vi "prueba_bloques.vi"() -> ()   [LabVIEW 2019]
uses:
  <vilib>/imath/engines/lvmath2/RunTimeEngine/Managers/WorkSpace/UID Generator.vi
  <vilib>/imath/engines/lvmath2/RunTimeEngine/IndexRead/NIMS V(S).vi
  <instcachedir>/0/NIMS V(S)_0488751826AF41519A22953C041130DC.lvgen/NIMS V(S)_0488751826AF41519A22953C041130DC_000.vi
  <vilib>/imath/engines/lvmath2/RunTimeEngine/BuiltInFunctions/atan2/NIMS_atan2.vi
  <instcachedir>/0/NIMS_atan2_A91AA4A7D42247EDBE8F76DB99AF04A4.lvgen/NIMS_atan2_A91AA4A7D42247EDBE8F76DB99AF04A4_000.vi
  <vilib>/imath/engines/lvmath2/RunTimeEngine/ErrorHandling/NIMS_Create Error From Enums.vi
  <vilib>/imath/engines/lvmath2/RunTimeEngine/ArithmeticOperatorToken/NIMS_ArithmeticOperator_power(S).vi
  <instcachedir>/0/NIMS_ArithmeticOperator_power(S)_F1497A2DE3CE4E82B2C3646D59904248.lvgen/NIMS_ArithmeticOperator_power(S)_F1497A2DE3CE4E82B2C3646D59904248_010.vi
  <vilib>/imath/engines/lvmath2/RunTimeEngine/BuiltInFunctions/acos/NIMS_acos(C).vi
  <instcachedir>/0/NIMS_acos(C)_835262ADAFAC4BBF9DF1C2958A624AC3.lvgen/NIMS_acos(C)_835262ADAFAC4BBF9DF1C2958A624AC3_001.vi
  <vilib>/imathl/engines/lvmath/Functions/Error Handling/Create Error.vi
  <vilib>/imath/engines/lvmath2/RunTimeEngine/RunTimeType/NIMS_RunTimeType_From StrictType (excl LVString).vi
  <instcachedir>/0/NIMS_RunTimeType_From StrictType (excl LVString)_D8AFBA86A94845AAA577C895450664BD.lvgen/NIMS_RunTimeType_From StrictType (excl LVString)_D8AFBA86A94845AAA577C895450664BD_000.vi
  <vilib>/imath/engines/lvmath2/RunTimeEngine/LocalVariableDefStatement/MC_LocalVariableDefStatement_Display.vi
  <vilib>/imath/engines/lvmath2/RunTimeEngine/RangeToken/NIMS_Range_R3 - Integer.vi
  <instcachedir>/0/NIMS_Range_R3 - Integer_E6E7B420460D4F08A65C42474AF91D7C.lvgen/NIMS_Range_R3 - Integer_E6E7B420460D4F08A65C42474AF91D7C_000.vi
  <vilib>/imath/engines/lvmath2/RunTimeEngine/CommandStatement/MC_CommandStatement_break.vi
  <vilib>/imath/engines/lvmath2/RunTimeEngine/VariableToken/NIMS_VariableToken_CondDefinedDefinedByReplace.vi
  <instcachedir>/0/NIMS_VariableToken_CondDefinedDefinedByReplace_D162CFFC24174562A9FEA619A91E1A56.lvgen/NIMS_VariableToken_CondDefinedDefinedByReplace_D162CFFC24174562A9FEA619A91E1A56_000.vi
  <vilib>/imath/engines/lvmath2/RunTimeEngine/IndexReplace/NIMS V(S)=S.vi
  <instcachedir>/0/NIMS V(S)=S_BD5C8CB81B6E4D99B8C0034EA1BEE55D.lvgen/NIMS V(S)=S_BD5C8CB81B6E4D99B8C0034EA1BEE55D_001.vi
  <vilib>/imath/engines/lvmath2/RunTimeEngine/VariableToken/NIMS_VariableToken_CondDefined.vi
  <instcachedir>/0/NIMS_VariableToken_CondDefined_30C3C94EAC01413DA882E848DEC89944.lvgen/NIMS_VariableToken_CondDefined_30C3C94EAC01413DA882E848DEC89944_000.vi
  <vilib>/imath/engines/lvmath/Functions/Error Handling/MergeErrorsWrapper.vi
  <vilib>/imath/engines/lvmath2/RunTimeEngine/Managers/SymbolTable/Clear UID.vi
  <vilib>/imath/engines/lvmath2/RunTimeEngine/NodeEndStatement/NIMS_NodeEndStatement_Output.vi
  <instcachedir>/0/NIMS_NodeEndStatement_Output_53EC0D466D134D7ABD903AC30B43404B.lvgen/NIMS_NodeEndStatement_Output_53EC0D466D134D7ABD903AC30B43404B_005.vi
  <instcachedir>/0/NIMS_NodeEndStatement_Output_53EC0D466D134D7ABD903AC30B43404B.lvgen/NIMS_NodeEndStatement_Output_53EC0D466D134D7ABD903AC30B43404B_009.vi
  <instcachedir>/0/NIMS_NodeEndStatement_Output_53EC0D466D134D7ABD903AC30B43404B.lvgen/NIMS_NodeEndStatement_Output_53EC0D466D134D7ABD903AC30B43404B_001.vi
  <instcachedir>/0/NIMS_NodeEndStatement_Output_53EC0D466D134D7ABD903AC30B43404B.lvgen/NIMS_NodeEndStatement_Output_53EC0D466D134D7ABD903AC30B43404B_000.vi
  <vilib>/imath/engines/lvmath2/RunTimeEngine/ErrorHandling/NIMS_Finalize Error.vi
  <vilib>/imath/engines/lvmath2/RunTimeEngine/Managers/SymbolTable/NIMS_WorkSpace.lvlib
panel:
  in  "Boolean":bool
  out "Waveform Chart 4":dbl(graph)
  out "Numeric 12":dbl format="%_7g"
  out "Numeric 11":dbl format="%_7g"
  out "Numeric 10":dbl format="%_7f"
  out "Numeric 9":dbl format="%_7g"
  out "Numeric 8":dbl format="%_7g"
  out "Numeric 7":dbl format="%_7g"
  out "Numeric 6":dbl format="%_7g"
  out "Numeric 5":dbl
  out "Waveform Chart 2":dbl(graph)
  in  "Tf":dbl
  in  "Y":dbl
  in  "X":dbl
  in  "stop":bool
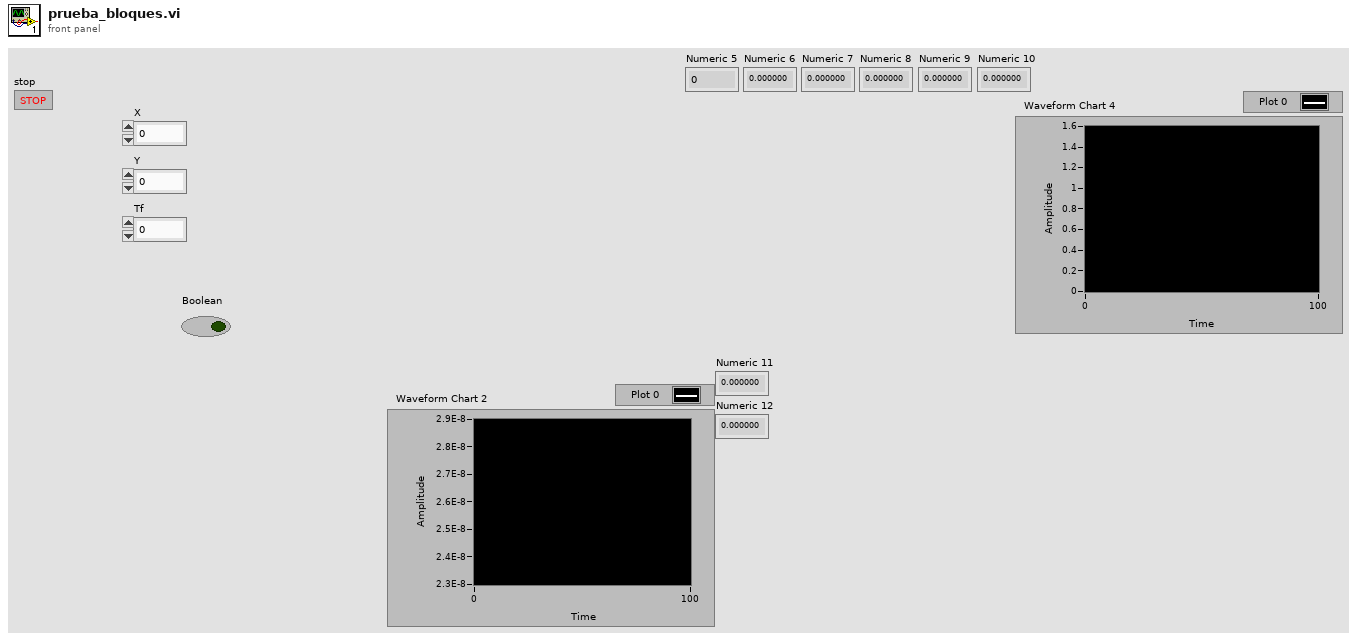
[diagram p1: front panel]
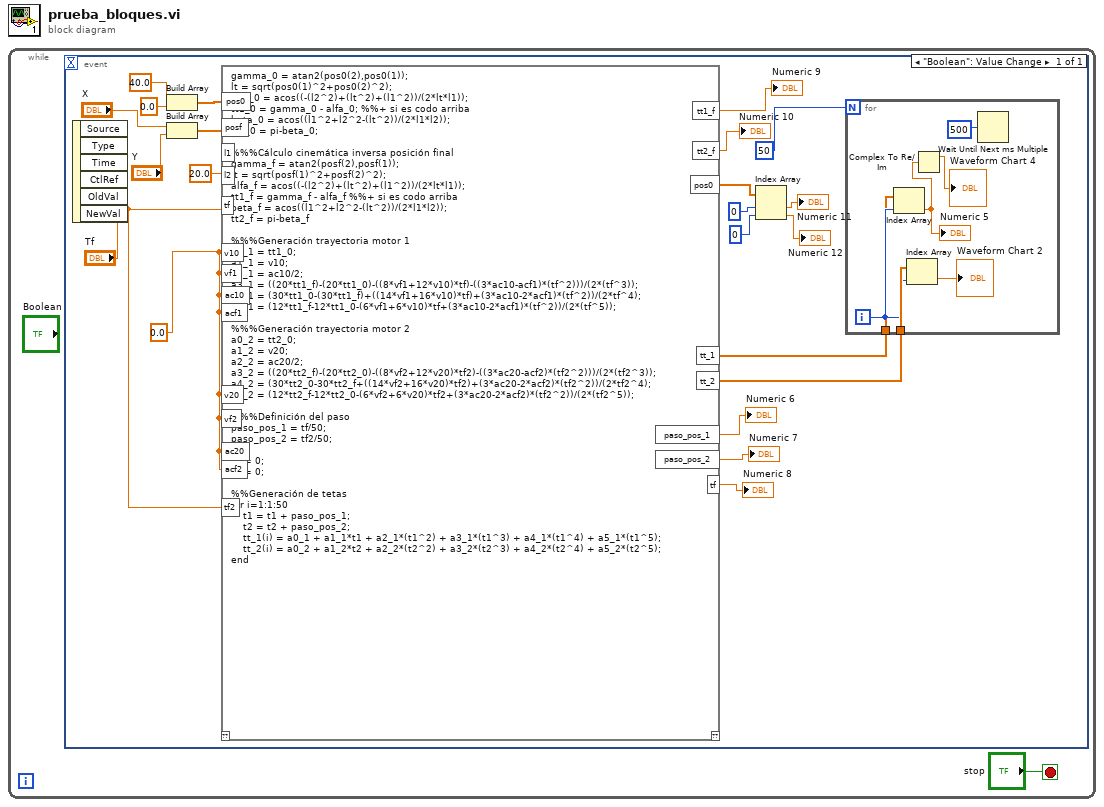
[diagram p0: block diagram]
diagram:
  n1 = while {
    stop <- "stop" stop-if-true
    n2 = event shown="[0] \"Boolean\": Value Change" {
      selector: _ -> [_]
      dyn-events: _ -> [_]
      timeout: _ -> [_]
      event "Boolean": Value Change {
        w19 = 0.0
        w23 = 20.0
        n3 = event-data() -> ()  [unwired: 1 in, 6 out]
        n4 = Build Array(40.0, 0.0) -> (w21:dbl[])
        n5 = Build Array("X", "Y") -> (w20:dbl[])
        n6 = mathscript code="gamma_0 = atan2(pos0(2),pos0(1));\nlt = sqrt(pos0(1)^2+pos0(2)^2);\nalfa_0 = acos((-(l2^2)+(lt^2)+(l1^2))/(2*lt*l1));\ntt1_0 = gamma_0 - alfa_0; %%+ si es codo arriba\nbeta_0 = acos((l1^2+l2^2-(lt^2))/(2*l1*l2));\ntt2_0 = pi-beta_0;\n\n%%%Cálculo cinemática inversa posición final\ngamma_f = atan2(posf(2),posf(1));\nlt = sqrt(posf(1)^2+posf(2)^2);\nalfa_f = acos((-(l2^2)+(lt^2)+(l1^2))/(2*lt*l1));\ntt1_f = gamma_f - alfa_f %%+ si es codo arriba\nbeta_f = acos((l1^2+l2^2-(lt^2))/(2*l1*l2));\ntt2_f = pi-beta_f\n\n%%%Generación trayectoria motor 1\na0_1 = tt1_0;\na1_1 = v10;\na2_1 = ac10/2;\na3_1 = ((20*tt1_f)-(20*tt1_0)-((8*vf1+12*v10)*tf)-((3*ac10-acf1)*(tf^2)))/(2*(tf^3));\na4_1 = (30*tt1_0-(30*tt1_f)+((14*vf1+16*v10)*tf)+(3*ac10-2*acf1)*(tf^2))/(2*tf^4);\na5_1 = (12*tt1_f-12*tt1_0-(6*vf1+6*v10)*tf+(3*ac10-2*acf1)*(tf^2))/(2*(tf^5));\n\n%%%Generación trayectoria motor 2\na0_2 = tt2_0;\na1_2 = v20;\na2_2 = ac20/2;\na3_2 = ((20*tt2_f)-(20*tt2_0)-((8*vf2+12*v20)*tf2)-((3*ac20-acf2)*(tf2^2)))/(2*(tf2^3));\na4_2 = (30*tt2_0-30*tt2_f+((14*vf2+16*v20)*tf2)+(3*ac20-2*acf2)*(tf2^2))/(2*tf2^4);\na5_2 = (12*tt2_f-12*tt2_0-(6*vf2+6*v20)*tf2+(3*ac20-2*acf2)*(tf2^2))/(2*(tf2^5));\n\n%%%Definición del paso\npaso_pos_1 = tf/50;\npaso_pos_2 = tf2/50;\n\nt1 = 0;\nt2 = 0;\n\n%%Generación de tetas\nfor i=1:1:50\n    t1 = t1 + paso_pos_1;\n    t2 = t2 + paso_pos_2;\n    tt_1(i) = a0_1 + a1_1*t1 + a2_1*(t1^2) + a3_1*(t1^3) + a4_1*(t1^4) + a5_1*(t1^5);\n    tt_2(i) = a0_2 + a1_2*t2 + a2_2*(t2^2) + a3_2*(t2^3) + a4_2*(t2^4) + a5_2*(t2^5);\nend"("pos0"=w21, "posf"=w20, "l1"=w23, "l2"=w23, "tf"="Tf", "v10"=w19, "vf1"=w19, "ac10"=w19, "acf1"=w19, "tf2"="Tf", "v20"=w19, "ac20"=w19, "vf2"=w19, "acf2"=w19) -> ("tt_1"=w2:cdb[], "tt_2"=w16:cdb[], "paso_pos_1"=→"Numeric 6":dbl, "paso_pos_2"=→"Numeric 7":dbl, "tf"=→"Numeric 8":dbl, "tt1_f"=→"Numeric 9":cdb, "tt2_f"=→"Numeric 10":cdb, "pos0"=w8:dbl[])  [unwired: 1 in, 1 out]
        n7 = Index Array(array=w8, index #1=0, index #2=0) -> (element #1=→"Numeric 11":dbl, element #2=→"Numeric 12":dbl)
        n8 = for {
          N: 50 -> [_]
          tunnel: w16 -> [w29]
          tunnel: w2 -> [w26]
          i -> [w27]
          n9 = Index Array(array=w26, index=w27) -> (element=w24:cdb)
          "Numeric 5" <- w24
          n10 = Index Array(array=w29, index=w27) -> (element=→"Waveform Chart 2":cdb)
          n11 = Complex To Re/Im(x + iy=w24) -> (x=→"Waveform Chart 4":dbl)  [unwired: 1 out]
          n12 = Wait Until Next ms Multiple(millisecond multiple=500) -> ()  [unwired: 1 out]
        }
      }
    }
  }
